vi "DAQmx.44xx.MIN MAX Fs.vi"(8 "error in (no error)":errorcluster) -> (0 "error out":errorcluster, 1 "Max(SampClk.MinRate) (S/s)":dbl, 2 "Min(SampClk.MaxRate) (S/s)":dbl)   [LabVIEW 2019, in "DAQmx.lvclass"]
doc: "Calculates the smallest maximum sample rate among all synchronized devices"
uses:
  DAQmx.lvclass
  <resource>/objmgr/daqmx.rc
panel:
  out "Fs (S/s)":dbl[](array[numeric]) format="%#_13g"
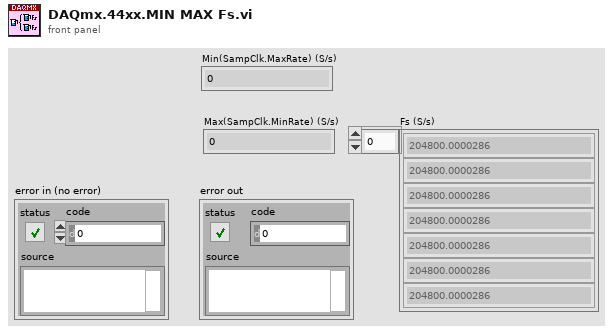
[diagram p1: front panel]
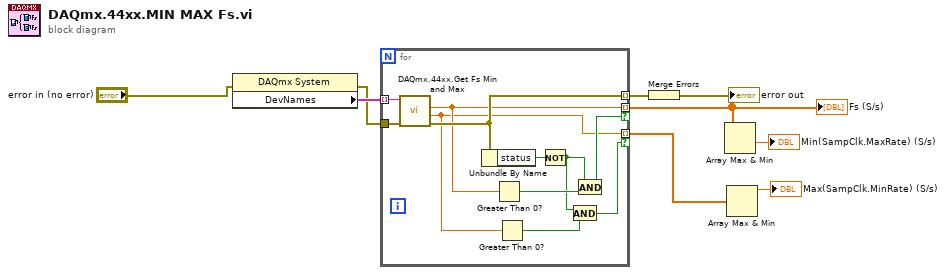
[diagram p0: block diagram]
diagram:
  n1 = property class="DAQmx System"(error in="error in (no error)") -> (error out=w2:errorcluster, "DevNames"=w3:tag[])  [unwired: 1 in, 1 out]
  n2 = for {
    tunnel: w3 -> [w20] mode=indexing
    tunnel: w2 -> [w19]
    tunnel: [w14] -> w4 mode=indexing if=w16
    tunnel: [w15] -> w1 mode=indexing
    tunnel: [w11] -> w6 mode=indexing if=w10
    n3 = call "DAQmx.44xx.Get Fs Min and Max.vi"("error in (no error)"=w19, "DAQmx Device Name"=w20) -> ("error out"=w15:errorcluster, "Fs Min"=w11:dbl, "Fs Max"=w14:dbl)  [unwired: 7 in]
    n4 = Unbundle By Name(w15) -> ("status"=w18:bool)
    n5 = Greater Than 0?(x=w14) -> (x > 0?=w17:bool)
    n6 = Greater Than 0?(x=w11) -> (x > 0?=w13:bool)
    n7 = Not(x=w18) -> (.not. x?=w12:bool)
    n8 = And(x=w12, y=w13) -> (x .and. y?=w10:bool)
    n9 = And(x=w12, y=w17) -> (x .and. y?=w16:bool)
  }
  "Fs (S/s)" <- w4
  n10 = Merge Errors(w1) -> (→"error out":errorcluster)
  n11 = Array Max & Min(array=w4) -> (min value=→"Min(SampClk.MaxRate) (S/s)":dbl)  [unwired: 3 out]
  n12 = Array Max & Min(array=w6) -> (max value=→"Max(SampClk.MinRate) (S/s)":dbl)  [unwired: 3 out]
